vi "Send Doodle coordinates.vi"(8 "error in":errorcluster, 9 "Row":u16, 10 "Col":u16, 11 "FPGA VI Reference Out":T1) -> (0 "error out":errorcluster, 3 "FPGA VI Reference Out 2":T1)   [LabVIEW 2019]
uses:
  TypeDefs/FPGA Reference.ctl
  <vilib>/Utility/error.llb/Error Cluster From Error Code.vi
  <vilib>/rvi/errors/niLvFpgaAdjustHostInterfaceError.vi
  <vilib>/rvi/interface/nirviReadWriteControl/nirviReadWriteControl.xnode
  FPGA Bitfiles/adafruitlcdsom_FPGATarget_FPGAMain_K7l+4zj6vFY.lvbitx
  FPGA Main.vi
  <vilib>/rvi/interface/nirviMethod/nirviMethod.xnode
  <vilib>/FPGAPlugInAG/sbRIO-9651/niLvFpga_WriteFifo_sbRIO-9651.vi
  <vilib>/rvi/errors/niLvFpgaMergeErrorWithErrorCode.vi
  NiFpgaLv.dll
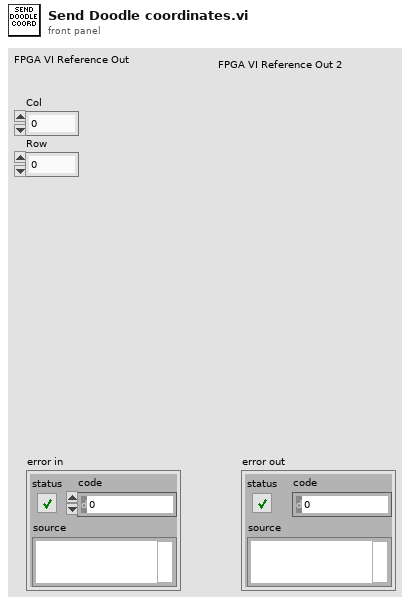
[diagram p1: front panel]
types:
  T1 = typedef "FPGA Reference.ctl" = refnum<k20>
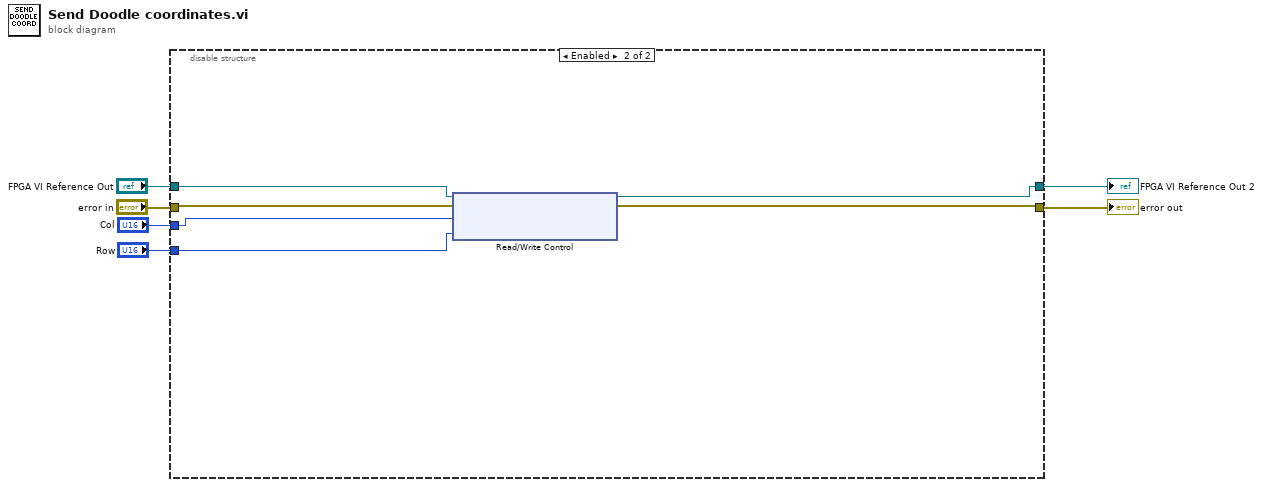
[diagram p0: block diagram]
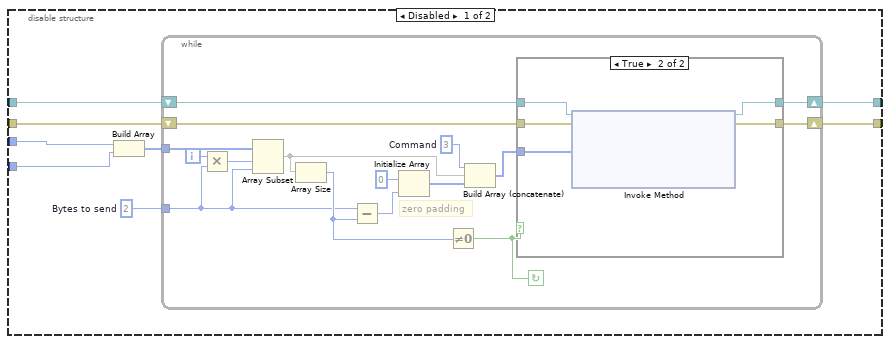
[diagram p2: hidden frame]
diagram:
  n1 = disable-structure shown="Enabled" {
    disable-tunnel: "FPGA VI Reference Out" -> [w14 w43]
    disable-tunnel: [w13 w40] -> w5
    disable-tunnel: [w12 w41] -> w4
    disable-tunnel: "error in" -> [w10 w42]
    disable-tunnel: "Col" -> [w9 w39]
    disable-tunnel: "Row" -> [w8 w38]
    frame Disabled {
      w11 = 2  # Bytes to send
      n2 = Build Array(w9, w8) -> (w7:u16[])
      n3 = while {
        shift-right: [w29] -> w13
        shift-left: w14 -> [w30]
        shift-right: [w28] -> w12
        shift-left: w10 -> [w27]
        tunnel: w7 -> [w24]
        tunnel: w11 -> [w15]
        i -> [w23]
        stop <- w18 continue-if-true
        w26 = u16 3  # Command
        # "zero padding"
        n4 = Multiply(x=w23, y=w15) -> (x*y=w22:i32)
        n5 = Array Subset(array=w24, index=w22, length=w15) -> (w21:u16[])
        n6 = Array Size(array=w21) -> (size(s)=w17:i32)
        n7 = Subtract(x=w15, y=w17) -> (x-y=w16:i32)
        n8 = Initialize Array(u16 0 ("X"), w16) -> (w19:u16[])
        n9 = Not Equal To 0?(x=w17) -> (x != 0?=w18:bool)
        n10 = Build Array (concatenate)(w26, w21, w19) -> (w25:u16[])
        n11 = case shown="True" w18 {
          tunnel: w30 -> [w32 w37]
          tunnel: [w32 w36] -> w29
          tunnel: [w31 w35] -> w28
          tunnel: w27 -> [w31 w34]
          tunnel: w25 -> [_ w33]
          frame False {
          }
          frame True {
            n12 = xnode "Invoke Method"("FPGA VI Reference In"=w37, "error in"=w34, "Data"=w33) -> ("FPGA VI Reference Out"=w36:T1, "error out"=w35:errorcluster)  [unwired: 1 in, 1 out]
          }
        }
      }
    }
    frame Enabled {
      n13 = xnode "Read/Write Control"("FPGA VI Reference In"=w43, "error in"=w42, "Col"=w39, "Row"=w38) -> ("FPGA VI Reference Out"=w40:T1, "error out"=w41:errorcluster)
    }
  }
  "FPGA VI Reference Out 2" <- w5
  "error out" <- w4
